vi "Read Bytes by Reference.vi"(8 "Error In":errorcluster, 10 "Count":u64, 11 "Reader In":refnum<data-value>) -> (0 "Error Out":errorcluster, 2 "Bytes":u8[](array[numeric]), 3 "Reader Out":refnum<data-value>)   [LabVIEW 2019, in "LabPack.lvlib" / "Reader.lvclass"]
uses:
  Reader.lvclass
  Reader.lvclass/Reader.ctl
  Handle Error.vi
  Public/Status/Read Status.vi
  Public/Status/Read Status Message.vi
  Public/Status/Read Is Error.vi
  Utility/Status Code.vi
  <vilib>/Utility/error.llb/Error Cluster From Error Code.vi
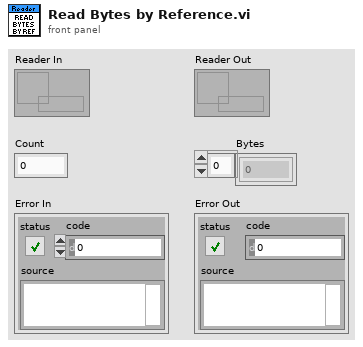
[diagram p1: front panel]
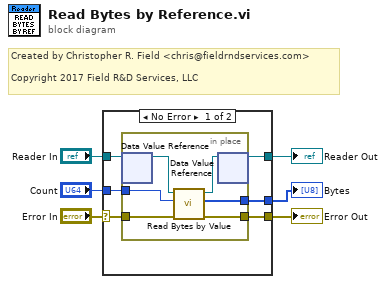
[diagram p0: block diagram]
diagram:
  # "Created by Christopher R. Field <chris@fieldrndservices.com>\n\nCopyright 2017 Field R&D Services, LLC"
  n1 = case shown="No Error" "Error In" {
    selector: "Error In" -> [w10 w19]
    tunnel: "Reader In" -> [w12 w20]
    tunnel: [w11 w20] -> w5
    tunnel: [w9 w19] -> w3
    tunnel: "Count" -> [w8 _]
    tunnel: [w7 _] -> w1
    frame No Error {
      n2 = in-place {
        in-place-border: w10 -> [w16]
        in-place-border: [w15] -> w9
        in-place-border: w8 -> [w14]
        in-place-border: [w13] -> w7
        n3 = in-place-dvr #1(w12) -> (w18:refnum<class "Reader.lvclass">)  [unwired: 1 out]
        n4 = call "Read Bytes by Value.vi"("Error In"=w16, "Count"=w14, "Reader In"=w18) -> ("Error Out"=w15:errorcluster, "Bytes"=w13:u8[], "Reader Out"=w17:refnum<class "Reader.lvclass">)  [unwired: 6 in]
        n5 = in-place-dvr #1(w17) -> (w11:refnum<data-value>)  [unwired: 1 out]
      }
    }
    frame Error {
    }
  }
  "Reader Out" <- w5
  "Error Out" <- w3
  "Bytes" <- w1
